vi "ScaleandControlChapter11.vi"(11 "axis info":T1) -> (3 "String":string)   [LabVIEW 2010]
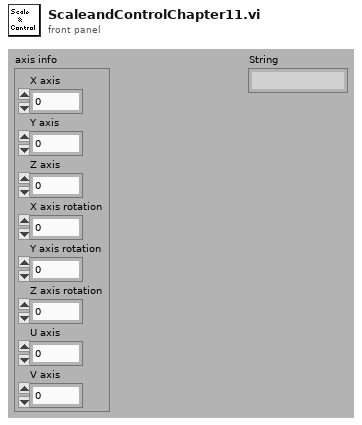
[diagram p1: front panel]
types:
  T1 = cluster{"X axis":i32, "Y axis":i32, "Z axis":i32, "X axis rotation":i32, "Y axis rotation":i32, "Z axis rotation":i32, "U axis":i32, "V axis":i32}
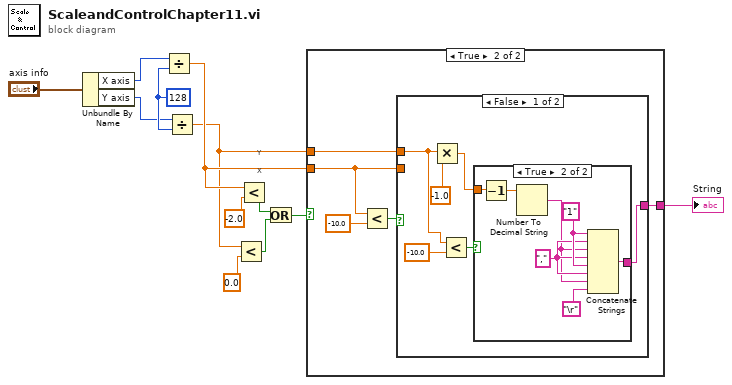
[diagram p0: block diagram]
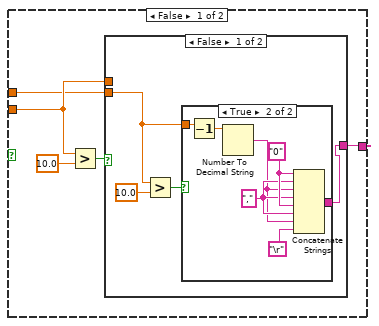
[diagram p2: hidden frame]
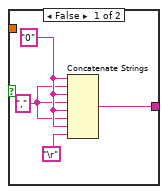
[diagram p3: hidden frame]
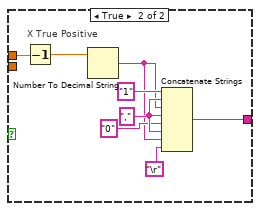
[diagram p4: hidden frame]
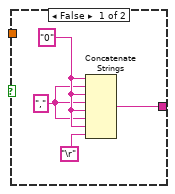
[diagram p5: hidden frame]
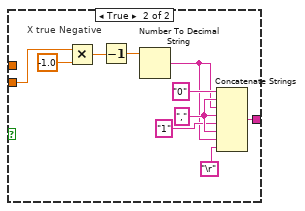
[diagram p6: hidden frame]
diagram:
  w7 = 128 ("y")
  # "X"
  # "Y"
  n1 = Unbundle By Name("axis info") -> ("X axis"=w5:i32, "Y axis"=w4:i32)
  n2 = Divide(x=w5, y=w7) -> (x/y=w10:dbl)
  n3 = Divide(x=w4, y=w7) -> (x/y=w3:dbl)
  n4 = Less?(x=w3, y=0.0) -> (x < y?=w9:bool)
  n5 = Less?(x=w10, y=-2.0) -> (x < y?=w12:bool)
  n6 = Or(x=w12, y=w9) -> (x .or. y?=w8:bool)
  n7 = case shown="True" w8 {
    tunnel: [w15 w43] -> w1
    tunnel: w10 -> [w14 w42]
    tunnel: w3 -> [w13 w41]
    frame False {
      n8 = Greater?(x=w14, y=10.0) -> (0:w17:bool)
      n9 = case shown="False" w17 {
        tunnel: [w19 w38] -> w15
        tunnel: w14 -> [_ w34]
        tunnel: w13 -> [w18 _]
        frame False {
          n10 = Greater?(x=w18, y=10.0) -> (0:w20:bool)
          n11 = case shown="True" w20 {
            tunnel: [w22 w29] -> w19
            tunnel: w18 -> [_ w27]
            frame False {
              w23 = "," ("string")
              w25 = "0" ("string")
              n12 = Concatenate Strings(w25, w23, w25, w23, w25, w23, w25, "\r") -> (w22:string)
            }
            frame True {
              w30 = "," ("string")
              w32 = "0" ("string")
              n13 = Decrement(x=w27) -> (x-1=w26:dbl)
              n14 = Number To Decimal String(number=w26) -> (decimal integer string=w28:string)  [unwired: 1 in]
              n15 = Concatenate Strings(w32, w30, w28, w30, w32, w30, w28, "\r") -> (w29:string)
            }
          }
        }
        frame True {
          w40 = "," ("string")
          # "X True Positive"
          n16 = Decrement(x=w34) -> (x-1=w33:dbl)
          n17 = Number To Decimal String(number=w33) -> (decimal integer string=w35:string)  [unwired: 1 in]
          n18 = Concatenate Strings("1" ("string"), w40, w35, w40, "0" ("string"), w40, w35, "\r") -> (w38:string)
        }
      }
    }
    frame True {
      n19 = Less?(x=w42, y=-10.0) -> (x < y?=w45:bool)
      n20 = case shown="False" w45 {
        tunnel: [w49 w69] -> w43
        tunnel: w42 -> [_ w65]
        tunnel: w41 -> [w46 _]
        frame False {
          n21 = Multiply(x=w46, y=-1.0) -> (x*y=w47:dbl)
          n22 = Less?(x=w46, y=-10.0) -> (x < y?=w50:bool)
          n23 = case shown="True" w50 {
            tunnel: [w52 w59] -> w49
            tunnel: w47 -> [_ w57]
            frame False {
              w53 = "," ("string")
              w55 = "0" ("string")
              n24 = Concatenate Strings(w55, w53, w55, w53, w55, w53, w55, "\r") -> (w52:string)
            }
            frame True {
              w60 = "," ("string")
              w62 = "1" ("string")
              n25 = Decrement(x=w57) -> (x-1=w56:dbl)
              n26 = Number To Decimal String(number=w56) -> (decimal integer string=w58:string)  [unwired: 1 in]
              n27 = Concatenate Strings(w62, w60, w58, w60, w62, w60, w58, "\r") -> (w59:string)
            }
          }
        }
        frame True {
          w72 = "," ("string")
          # "X true Negative"
          n28 = Multiply(x=w65, y=-1.0) -> (x*y=w64:dbl)
          n29 = Decrement(x=w64) -> (x-1=w63:dbl)
          n30 = Number To Decimal String(number=w63) -> (decimal integer string=w66:string)  [unwired: 1 in]
          n31 = Concatenate Strings("0" ("string"), w72, w66, w72, "1" ("string"), w72, w66, "\r") -> (w69:string)
        }
      }
    }
  }
  "String" <- w1
